vi "_HDBn.vi"(1 "输入":i8[](array[numeric]), 2 "n":dbl=3.0) -> (0 "输出":i8[](array[numeric]))   [LabVIEW 2018]
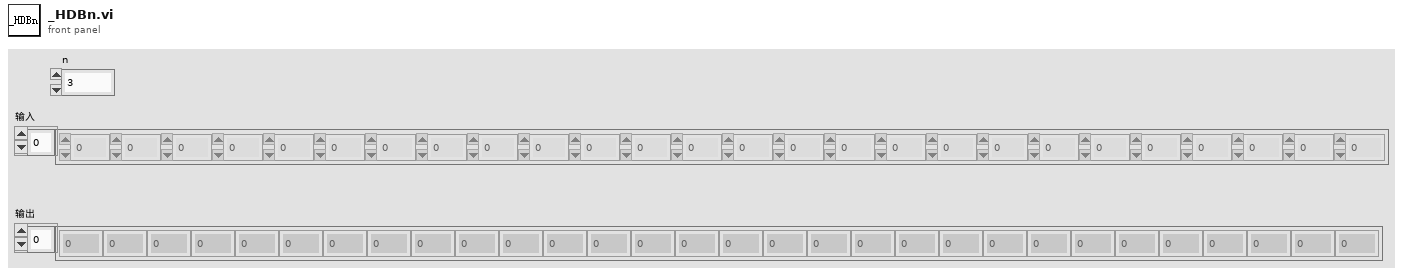
[diagram p1: front panel]
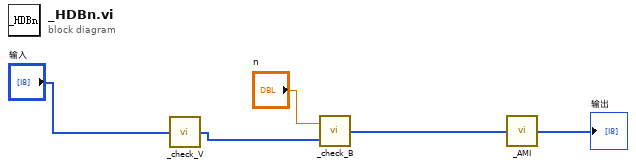
[diagram p0: block diagram]
diagram:
  n1 = call "_check_V.vi"("输入"="输入") -> ("输出"=w4:i8[])
  n2 = call "_check_B.vi"("输入"=w4, "n"="n") -> ("输出"=w2:i8[])
  n3 = call "_AMI.vi"("输入"=w2) -> ("输出"=→"输出":i8[])
